vi "ScaleGraphX (SubVI).vi"(9 "Array":dbl[](array[numeric]), 10 "Übersetzung ermitteln aus":u8, 11 "XYGraph (Eingang)":refnum<vi>) -> (0 "xMax (Ausgang)":dbl, 1 "xMin (Ausgang)":dbl)   [LabVIEW 2014]
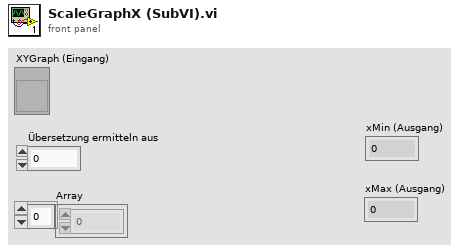
[diagram p1: front panel]
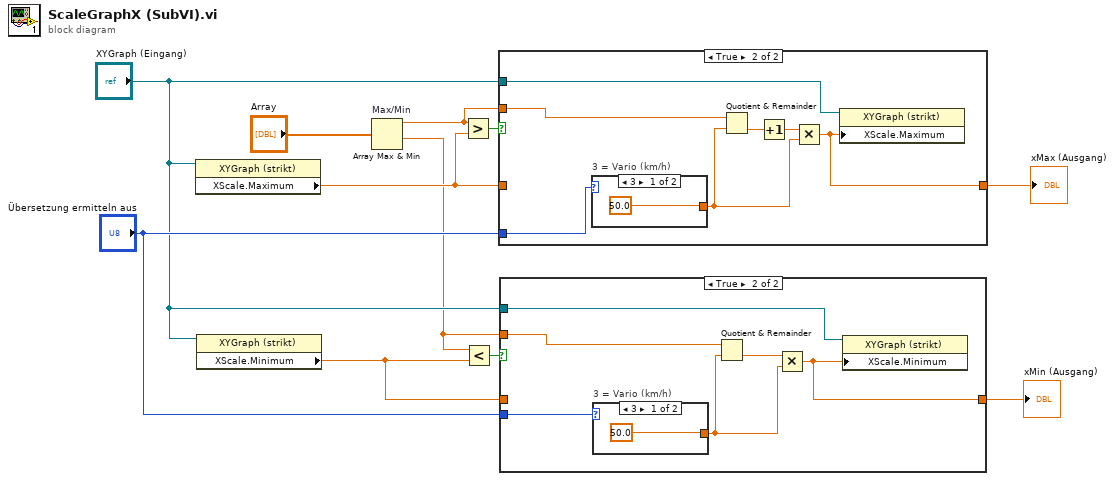
[diagram p0: block diagram]
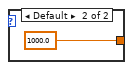
[diagram p3: hidden frame]
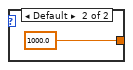
[diagram p5: hidden frame]
diagram:
  n1 = property on="Eigenschaftsknoten" class="XYGraph (strikt)"(reference="XYGraph (Eingang)") -> ("XScale.Maximum"=w4:dbl)  [unwired: 1 in, 2 out]
  n2 = property on="Eigenschaftsknoten" class="XYGraph (strikt)"(reference="XYGraph (Eingang)") -> ("XScale.Minimum"=w3:dbl)  [unwired: 1 in, 2 out]
  n3 = Array Max & Min "Max/Min"(array="Array") -> (max value=w1:dbl, min value=w2:dbl)  [unwired: 2 out]
  n4 = Greater?(x=w1, y=w4) -> (0:w10:bool)
  n5 = Less?(x=w2, y=w3) -> (x < y?=w9:bool)
  n6 = case shown="True" w10 {
    tunnel: "XYGraph (Eingang)" -> [_ w17]
    tunnel: "Übersetzung ermitteln aus" -> [_ w15]
    tunnel: [w12 w14] -> w6
    tunnel: w4 -> [w12 _]
    tunnel: w1 -> [_ w13]
    frame False {
    }
    frame True {
      n7 = case "3 = Vario (km/h)" shown="3" w15 {
        tunnel: [50.0 1000.0] -> w16
        frame 3 {
        }
        frame Default {
        }
      }
      n8 = Quotient & Remainder(x=w13, y=w16) -> (floor(x/y)=w18:dbl)  [unwired: 1 out]
      n9 = Increment(x=w18) -> (x+1=w19:dbl)
      n10 = Multiply(x=w19, y=w16) -> (x*y=w14:dbl)
      n11 = property on="Eigenschaftsknoten" class="XYGraph (strikt)"(reference=w17, "XScale.Maximum"=w14) -> ()  [unwired: 1 in, 2 out]
    }
  }
  "xMax (Ausgang)" <- w6
  n12 = case shown="True" w9 {
    tunnel: "XYGraph (Eingang)" -> [_ w28]
    tunnel: "Übersetzung ermitteln aus" -> [_ w26]
    tunnel: [w22 w24] -> w5
    tunnel: w3 -> [w22 _]
    tunnel: w2 -> [_ w23]
    frame False {
    }
    frame True {
      n13 = case "3 = Vario (km/h)" shown="3" w26 {
        tunnel: [50.0 1000.0] -> w27
        frame 3 {
        }
        frame Default {
        }
      }
      n14 = Quotient & Remainder(x=w23, y=w27) -> (floor(x/y)=w25:dbl)  [unwired: 1 out]
      n15 = Multiply(x=w25, y=w27) -> (x*y=w24:dbl)
      n16 = property on="Eigenschaftsknoten" class="XYGraph (strikt)"(reference=w28, "XScale.Minimum"=w24) -> ()  [unwired: 1 in, 2 out]
    }
  }
  "xMin (Ausgang)" <- w5
